vi "CubeStructure.vi"() -> (0 "cube structure array (8 corners)":cluster{T1, "element":T1, "element":T1}[](array[cluster]), 1 "cube structure array (12 edges)":cluster{T1, "element":T1}[](array[cluster]))   [LabVIEW 2017]
uses:
  FaceletID.ctl
  FaceSymbols.ctl
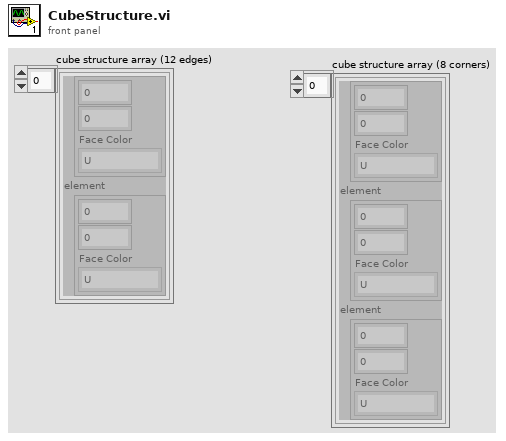
[diagram p1: front panel]
types:
  T1 = typedef "FaceletID.ctl" = cluster{i32, i32, "Face Color":T2}
  T2 = typedef "FaceSymbols.ctl" = enum16{"U", "L", "F", "R", "B", "D"}
  T3 = cluster{"element":T1, "element":T1, "element":T1}
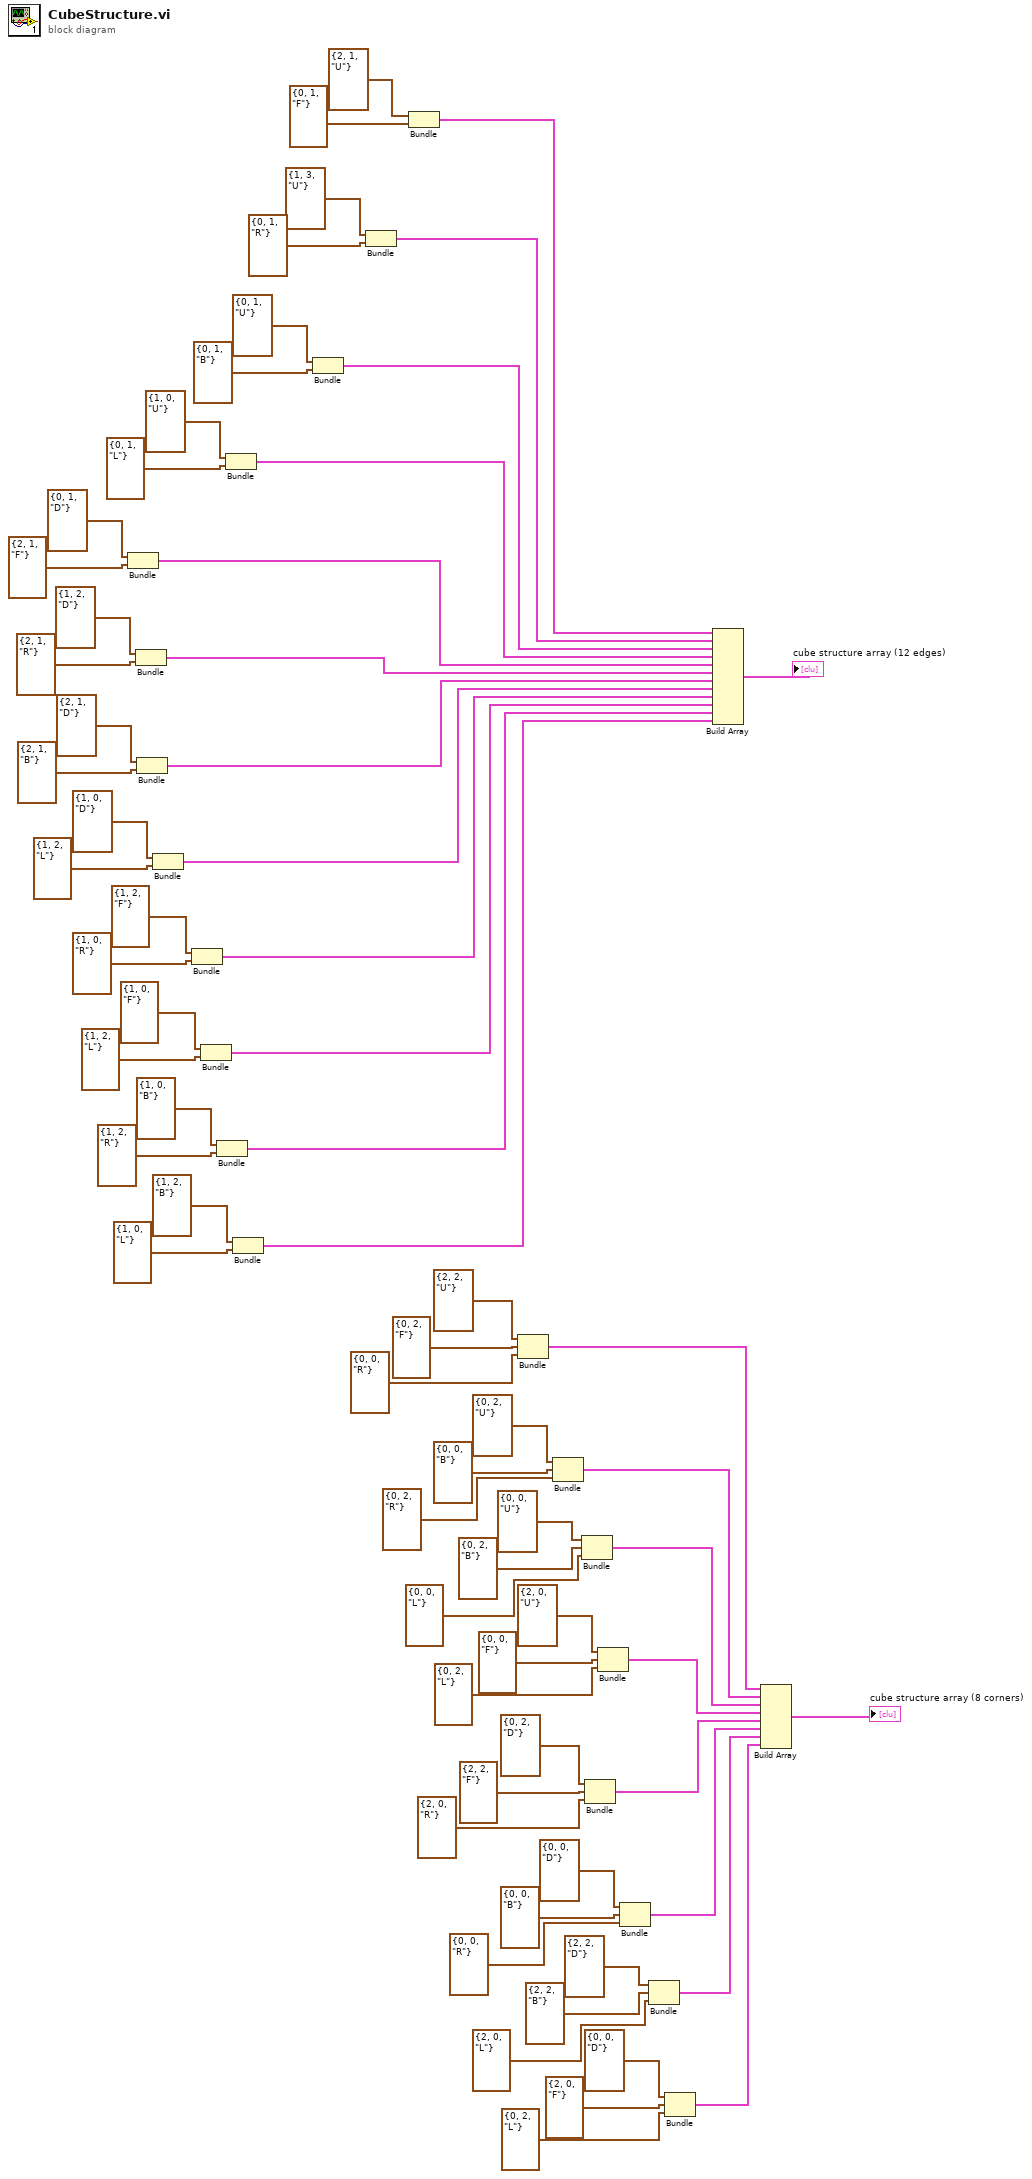
[diagram p0: block diagram]
diagram:
  n1 = Bundle(T1 {0, 1, "Face Color"=enum."D"}, "element"=T1 {2, 1, "Face Color"=enum."F"}) -> (w11:cluster{T1, "element":T1})  [unwired: 1 in]
  n2 = Bundle(T1 {1, 2, "Face Color"=enum."D"}, "element"=T1 {2, 1, "Face Color"=enum."R"}) -> (w12:cluster{T1, "element":T1})  [unwired: 1 in]
  n3 = Bundle(T1 {2, 1, "Face Color"=enum."D"}, "element"=T1 {2, 1, "Face Color"=enum."B"}) -> (w42:cluster{T1, "element":T1})  [unwired: 1 in]
  n4 = Bundle(T1 {1, 0, "Face Color"=enum."D"}, "element"=T1 {1, 2, "Face Color"=enum."L"}) -> (w41:cluster{T1, "element":T1})  [unwired: 1 in]
  n5 = Bundle(T1 {1, 2, "Face Color"=enum."F"}, "element"=T1 {1, 0, "Face Color"=enum."R"}) -> (w40:cluster{T1, "element":T1})  [unwired: 1 in]
  n6 = Bundle(T1 {1, 0, "Face Color"=enum."F"}, "element"=T1 {1, 2, "Face Color"=enum."L"}) -> (w39:cluster{T1, "element":T1})  [unwired: 1 in]
  n7 = Bundle(T1 {1, 0, "Face Color"=enum."B"}, "element"=T1 {1, 2, "Face Color"=enum."R"}) -> (w38:cluster{T1, "element":T1})  [unwired: 1 in]
  n8 = Bundle(T1 {1, 0, "Face Color"=enum."U"}, "element"=T1 {0, 1, "Face Color"=enum."L"}) -> (w37:cluster{T1, "element":T1})  [unwired: 1 in]
  n9 = Bundle(T1 {1, 2, "Face Color"=enum."B"}, "element"=T1 {1, 0, "Face Color"=enum."L"}) -> (w36:cluster{T1, "element":T1})  [unwired: 1 in]
  n10 = Bundle(T1 {0, 1, "Face Color"=enum."U"}, "element"=T1 {0, 1, "Face Color"=enum."B"}) -> (w61:cluster{T1, "element":T1})  [unwired: 1 in]
  n11 = Bundle(T1 {1, 3, "Face Color"=enum."U"}, "element"=T1 {0, 1, "Face Color"=enum."R"}) -> (w65:cluster{T1, "element":T1})  [unwired: 1 in]
  n12 = Bundle(T1 {2, 1, "Face Color"=enum."U"}, "element"=T1 {0, 1, "Face Color"=enum."F"}) -> (w68:cluster{T1, "element":T1})  [unwired: 1 in]
  n13 = Bundle("element"=T1 {2, 2, "Face Color"=enum."U"}, "element"=T1 {0, 2, "Face Color"=enum."F"}, "element"=T1 {0, 0, "Face Color"=enum."R"}) -> (w10:T3)  [unwired: 1 in]
  n14 = Bundle(T1 {0, 2, "Face Color"=enum."U"}, "element"=T1 {0, 0, "Face Color"=enum."B"}, "element"=T1 {0, 2, "Face Color"=enum."R"}) -> (w9:cluster{T1, "element":T1, "element":T1})  [unwired: 1 in]
  n15 = Bundle(T1 {0, 0, "Face Color"=enum."U"}, "element"=T1 {0, 2, "Face Color"=enum."B"}, "element"=T1 {0, 0, "Face Color"=enum."L"}) -> (w8:cluster{T1, "element":T1, "element":T1})  [unwired: 1 in]
  n16 = Bundle("element"=T1 {0, 2, "Face Color"=enum."D"}, "element"=T1 {2, 2, "Face Color"=enum."F"}, "element"=T1 {2, 0, "Face Color"=enum."R"}) -> (w6:T3)  [unwired: 1 in]
  n17 = Bundle(T1 {2, 0, "Face Color"=enum."U"}, "element"=T1 {0, 0, "Face Color"=enum."F"}, "element"=T1 {0, 2, "Face Color"=enum."L"}) -> (w7:cluster{T1, "element":T1, "element":T1})  [unwired: 1 in]
  n18 = Bundle(T1 {0, 0, "Face Color"=enum."D"}, "element"=T1 {0, 0, "Face Color"=enum."B"}, "element"=T1 {0, 0, "Face Color"=enum."R"}) -> (w5:cluster{T1, "element":T1, "element":T1})  [unwired: 1 in]
  n19 = Bundle(T1 {2, 2, "Face Color"=enum."D"}, "element"=T1 {2, 2, "Face Color"=enum."B"}, "element"=T1 {2, 0, "Face Color"=enum."L"}) -> (w4:cluster{T1, "element":T1, "element":T1})  [unwired: 1 in]
  n20 = Bundle(T1 {0, 0, "Face Color"=enum."D"}, "element"=T1 {2, 0, "Face Color"=enum."F"}, "element"=T1 {0, 2, "Face Color"=enum."L"}) -> (w3:cluster{T1, "element":T1, "element":T1})  [unwired: 1 in]
  n21 = Build Array(w68, w65, w61, w37, w11, w12, w42, w41, w40, w39, w38, w36) -> (→"cube structure array (12 edges)":cluster{T1, "element":T1}[])
  n22 = Build Array(w10, w9, w8, w7, w6, w5, w4, w3) -> (→"cube structure array (8 corners)":cluster{T1, "element":T1, "element":T1}[])
